vi "Test To String on Non String Array.vi"(11 "Test Case In":refnum<class "Basic Mechanics Tests.lvclass">) -> (0 "error out":errorcluster, 3 "Test Case Out":refnum<class "Basic Mechanics Tests.lvclass">)   [LabVIEW 2020, in "Basic Mechanics Tests.lvclass"]
uses:
  Basic Mechanics Tests.lvclass
  C:/Program Files/National Instruments/LabVIEW 2026/vi.lib/Astemes/LUnit/Test Case.lvclass
  <vilib>/Astemes/LUnit/Test Case.lvclass/Test Case.ctl
  21842cc0-253c-4332-b0cc-dff950d5b8d1.vi
  4993e8ee-a06a-463a-9684-69129f64d5ce.vi
  21842cc0-253c-4332-b0cc-dff950d5b8d1.vi/5b84c07b-8b36-46ce-878d-0b3558e12aa4.vi
  <vilib>/Astemes/LUnit/Core/LUnit Test Case/Private/Append Pass Result.vi
  <vilib>/Astemes/LUnit/Core/LUnit Test Case/Private/Append Fail Result.vi
  4993e8ee-a06a-463a-9684-69129f64d5ce.vi/9c5d11cd-9439-4240-a1ee-d9baace9c924.vi
  21842cc0-253c-4332-b0cc-dff950d5b8d1.vi/5b84c07b-8b36-46ce-878d-0b3558e12aa4.vi/b30c0498-5c87-4a37-a7a8-8ea35c3fd313.vi
  <vilib>/Astemes/LUnit/Core/LUnit Test Case/Private/Run In UI.vi
  <vilib>/Utility/error.llb/Clear Errors.vi
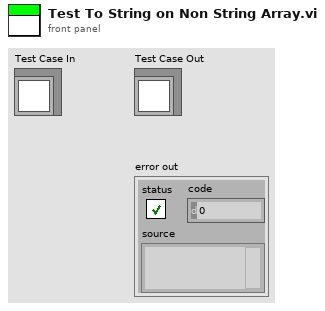
[diagram p1: front panel]
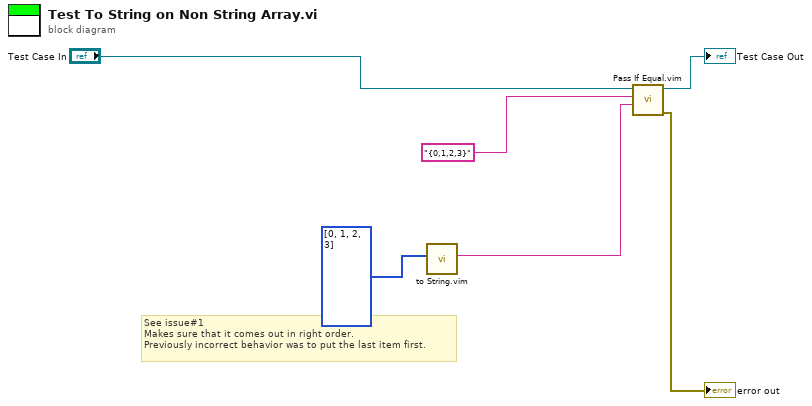
[diagram p0: block diagram]
diagram:
  # "See issue#1\nMakes sure that it comes out in right order.\nPreviously incorrect behavior was to put the last item first."
  n1 = call "to String.vim"("Anything"=i32[] [0, 1, 2, 3]) -> ("log string"=w2:string)  [unwired: 10 in]
  n2 = call "Pass If Equal.vim"("Actual"=w2, "Expected"="{0,1,2,3}" ("log string"), "LUnit Test Case In"="Test Case In") -> ("error out"=→"error out":errorcluster, "LUnit Test Case Out"=→"Test Case Out":refnum<class "Basic Mechanics Tests.lvclass">)  [unwired: 7 in]
